vi "Disconnect.vi"(8 "Error In":errorcluster, 11 "AMS Connection":T1) -> (0 "Error Out":errorcluster)   [LabVIEW 2019, in "TwinCAT ADS.lvlib"]
uses:
  <userlib>/PMA/TwinCAT ADS.lvlib
  <userlib>/PMA/Low Level/TypeDefs/AMS Connection.ctl
  <userlib>/PMA/Low Level/TypeDefs/AMS.ctl
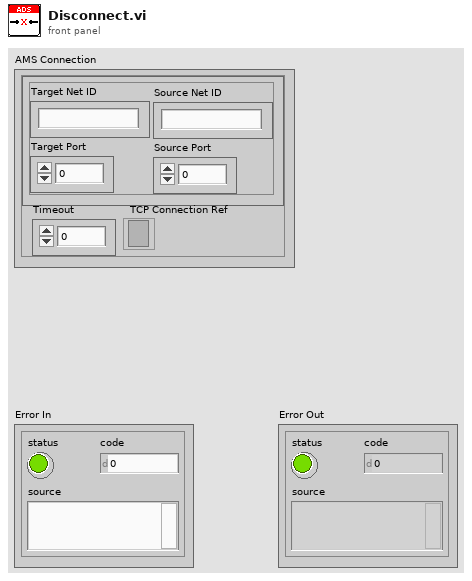
[diagram p1: front panel]
types:
  T1 = typedef "TwinCAT ADS.lvlib/AMS Connection.ctl" = cluster{"AMS":T2, "Timeout":i32, "TCP Connection Ref":refnum<k5>}
  T2 = typedef "TwinCAT ADS.lvlib/AMS.ctl" = cluster{"Target Net ID":string, "Target Port":u16, "Source Net ID":string, "Source Port":u16}
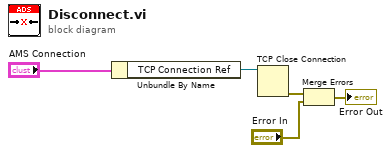
[diagram p0: block diagram]
diagram:
  n1 = Unbundle By Name("AMS Connection") -> ("TCP Connection Ref"=w4:refnum<k5>)
  n2 = TCP Close Connection(connection ID=w4) -> (error out=w2:errorcluster)  [unwired: 2 in, 1 out]
  n3 = Merge Errors(w2, "Error In") -> (→"Error Out":errorcluster)
